vi "Read Value (NT Base).vi"(8 "error in (no error)":errorcluster, 10 "default value":refnum<class "Base Interface.lvclass">, 11 "PV Data in":refnum<class "PV Data.lvclass">) -> (0 "error out":errorcluster, 2 "value":refnum<class "Base Interface.lvclass">, 3 "PV Data out":refnum<class "PV Data.lvclass">)   [LabVIEW 2020, in "PV Access.lvlib" / "PV Data.lvlib" / "PV Data.lvclass"]
uses:
  PV Data.lvclass
  Base Interface/Base Interface.lvclass
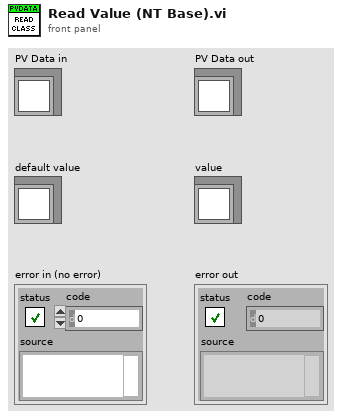
[diagram p1: front panel]
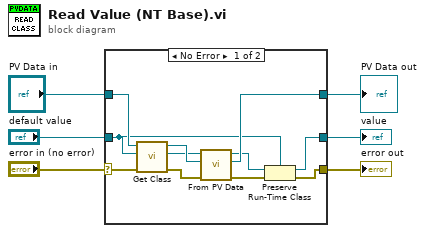
[diagram p0: block diagram]
diagram:
  n1 = case shown="No Error" "error in (no error)" {
    selector: "error in (no error)" -> [w14 w20]
    tunnel: [w10 w20] -> w5
    tunnel: [w15 w19] -> w3
    tunnel: "PV Data in" -> [w16 w19]
    tunnel: "default value" -> [w9 w18]
    tunnel: [w11 w18] -> w1
    frame No Error {
      n2 = call "Get Class.vi"("error in (no error)"=w14, "default"=w9, "PV Data in"=w16) -> ("error out"=w12:errorcluster, "Value out"=w13:refnum<class "Base Interface.lvclass">, "PV Data out"=w17:refnum<class "PV Data.lvclass">)  [unwired: 6 in]
      n3 = call-dynamic "From PV Data.vi"("error in"=w12, "PV data in"=w17, "Base Interface in"=w13) -> ("error out"=w7:errorcluster, "PV data out"=w15:refnum<class "PV Data.lvclass">, "Base Interface out"=w8:refnum<class "Base Interface.lvclass">)  [unwired: 6 in]
      n4 = Preserve Run-Time Class(object in=w8, error in=w7, 2:w9) -> (object out=w11:refnum<class "Base Interface.lvclass">, error out=w10:errorcluster)
    }
    frame Error {
    }
  }
  "error out" <- w5
  "PV Data out" <- w3
  "value" <- w1
